vi "testBatchInvalidElements.vi"(8 "error in (no error)":errorcluster, 11 "TestCase in":refnum<class "ServerTest.lvclass">) -> (0 "error out":errorcluster, 3 "TestCase out":refnum<class "ServerTest.lvclass">)   [LabVIEW 2017, in "ServerTest.lvclass"]
uses:
  ServerTest.lvclass
  <vilib>/addons/_JKI Toolkits/VI Tester/TestCase.llb/TestCase.lvclass
  C:/Program Files (x86)/National Instruments/LabVIEW 2017/vi.lib/addons/_JKI Toolkits/VI Tester/TestCase.llb/TestCase.lvclass
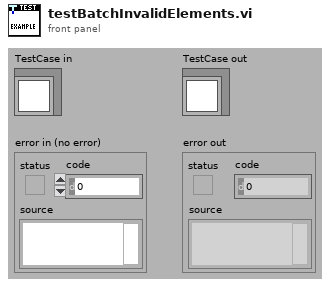
[diagram p1: front panel]
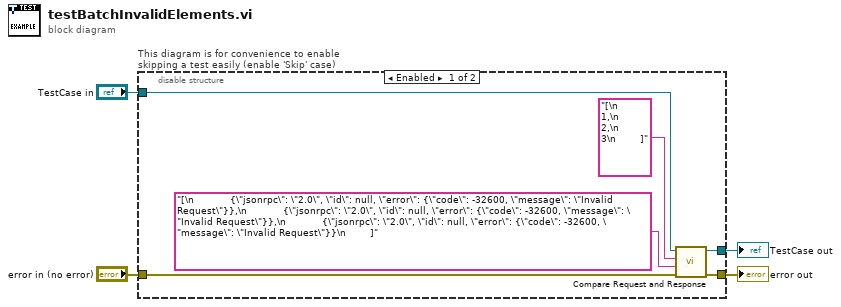
[diagram p0: block diagram]
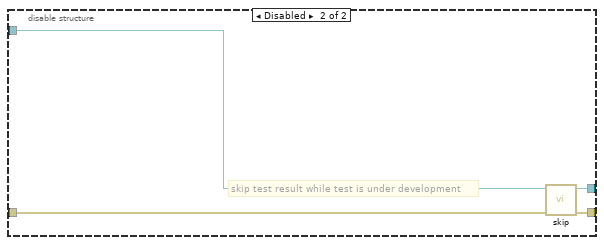
[diagram p2: hidden frame]
diagram:
  n1 = disable-structure "This diagram is for convenience to enable skipping a test easily (enable 'Skip' case)" shown="Enabled" {
    disable-tunnel: "TestCase in" -> [w8 w14]
    disable-tunnel: [w7 w12] -> w1
    disable-tunnel: [w9 w13] -> w3
    disable-tunnel: "error in (no error)" -> [w10 w11]
    frame Enabled {
      n2 = call "Compare Request and Response.vi"("error in (no error)"=w10, "JSON Response String"="[\n            {\"jsonrpc\": \"2.0\", \"id\": null, \"error\": {\"code\": -32600, \"message\": \"Invalid Request\"}},\n            {\"jsonrpc\": \"2.0\", \"id\": null, \"error\": {\"code\": -32600, \"message\": \"Invalid Request\"}},\n            {\"jsonrpc\": \"2.0\", \"id\": null, \"error\": {\"code\": -32600, \"message\": \"Invalid Request\"}}\n        ]", "JSON Request String"="[\n            1,\n            2,\n            3\n        ]", "ServerTest in"=w8) -> ("error out"=w9:errorcluster, "ServerTest out"=w7:refnum<class "ServerTest.lvclass">)  [unwired: 6 in]
    }
    frame Disabled {
      # "skip test result while test is under development"
      n3 = call <vilib>:"skip.vi"("error in (no error)"=w11, "TestCase in"=w14) -> ("error out"=w13:errorcluster, "TestCase out"=w12:refnum<class "ServerTest.lvclass">)  [unwired: 8 in]
    }
  }
  "error out" <- w3
  "TestCase out" <- w1
